vi "parse data file basename string.vi"(11 "base name":string="^[0-9]+") -> (3 "output cluster":T1, 4 "exact match":bool)   [LabVIEW 2012]
uses:
  <vilib>/regexp/Match Regular Expression.xnode
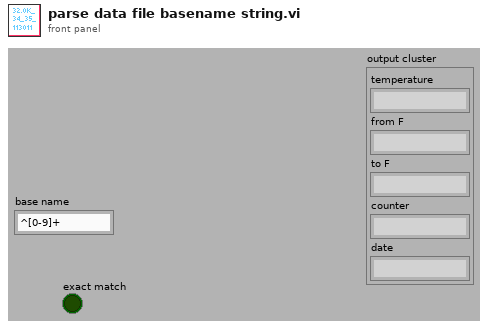
[diagram p1: front panel]
types:
  T1 = cluster{"temperature":string, "from F":string, "to F":string, "counter":string, "date":string}
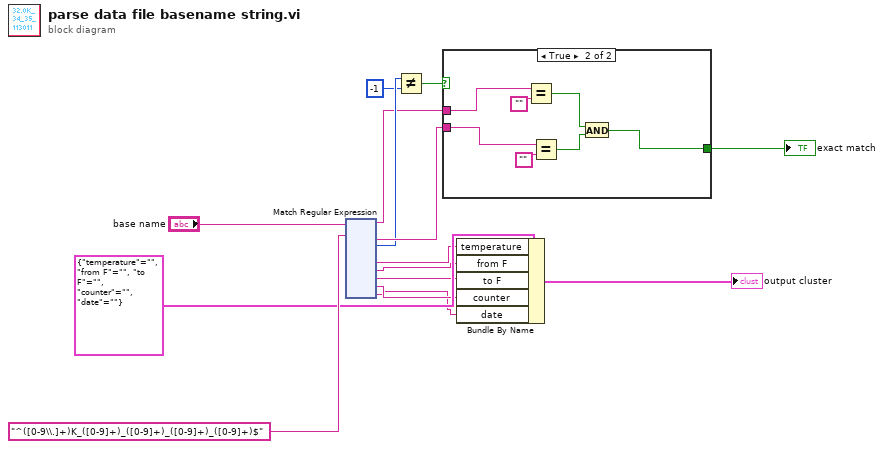
[diagram p0: block diagram]
diagram:
  n1 = xnode "Match Regular Expression"("input string"="base name", "regular expression"="^([0-9\\.]+)K_([0-9]+)_([0-9]+)_([0-9]+)_([0-9]+)$" ("string")) -> ("before match"=w12:string, "after match"=w15:string, "offset past match"=w14:i32, "submatch 1"=w6:string, "submatch 2"=w5:string, "submatch 3"=w4:string, "submatch 4"=w3:string, "submatch 5"=w2:string)  [unwired: 4 in, 2 out]
  n2 = Not Equal?(x=w14, y=-1) -> (x != y?=w11:bool)
  n3 = case shown="True" w11 {
    selector: w11 -> [w16 _]
    tunnel: w15 -> [_ w22]
    tunnel: w12 -> [_ w17]
    tunnel: [w16 w18] -> w10
    frame False {
    }
    frame True {
      n4 = Equal?(x=w17, y="") -> (x = y?=w19:bool)
      n5 = Equal?(x=w22, y="") -> (x = y?=w20:bool)
      n6 = And(x=w19, y=w20) -> (x .and. y?=w18:bool)
    }
  }
  "exact match" <- w10
  n7 = Bundle By Name(cluster=T1 {"temperature"="", "from F"="", "to F"="", "counter"="", "date"=""}, "temperature"=w6, "from F"=w5, "to F"=w4, "counter"=w3, "date"=w2) -> (→"output cluster":T1)
